vi "Default Settings.vi"() -> (0 "default settings":T1 {"Simulated Signal"."amplitude" format="%.0pV"; "Simulated Signal"."frequency" format="%.2pHz"; "input range" format="%.0pV"; "sample rate" format="%.2pHz"})   [LabVIEW 2019]
uses:
  Measure and Log Settings.ctl
  Simulated Signal Type.ctl
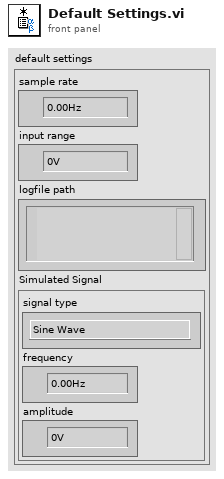
[diagram p1: front panel]
types:
  T1 = typedef "Measure and Log Settings.ctl" = cluster{"sample rate":dbl, "input range":dbl, "logfile path":path, "Simulated Signal":cluster{"signal type":T2, "frequency":dbl, "amplitude":dbl}}
  T2 = typedef "Simulated Signal Type.ctl" = enum16{"Sine Wave", "Square Wave with Noise"}
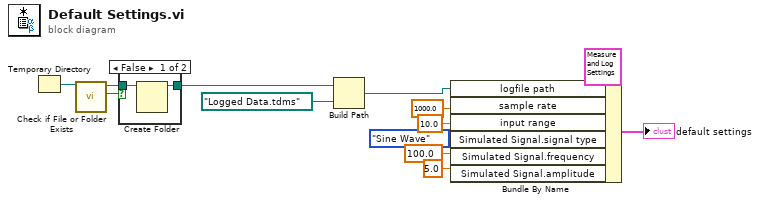
[diagram p0: block diagram]
diagram:
  n1 = Temporary Directory() -> (w12:path)
  n2 = call <vilib>:"Check if File or Folder Exists.vi"("path"=w12) -> ("file or folder exists?"=w9:bool, "dup path"=w10:path)  [unwired: 8 in, 1 out]
  n3 = case shown="False" w9 {
    tunnel: w10 -> [w15 w16]
    tunnel: [w14 w16] -> w11
    frame False {
      n4 = Create Folder(path (use dialog)=w15) -> (created path=w14:path)  [unwired: 2 in, 2 out]
    }
    frame True {
    }
  }
  n5 = Build Path(base path=w11, name or relative path=path "Logged Data.tdms" ("App:Default Data Directory")) -> (appended path=w13:path)
  n6 = Bundle By Name(cluster=T1 {"sample rate"=100.0, "input range"=10.0, "logfile path"=path "/Bohr/private/var/folders/6r/yp35wkn10pv4lxqxxk3gyl6h0000gq/T/TemporaryItems/Logged Data.tdms", "Simulated Signal"={"signal type"=enum."Sine Wave", "frequency"=1000.0, "amplitude"=5.0}} ("default settings"), "logfile path"=w13, "sample rate"=1000.0, "input range"=10.0, "Simulated Signal.signal type"=Simulated_Signal_Type."Sine Wave", "Simulated Signal.frequency"=100.0 ("sample rate"), "Simulated Signal.amplitude"=5.0 ("input range")) -> (→"default settings":T1)
